vi "Swerve_Wheel.vi"(3 "Kp":dbl, 4 "Offset_Y":dbl, 5 "Offset_X":dbl, 6 "Wheel_Angle":dbl, 7 "Z":dbl, 8 "Y":dbl, 9 "X":dbl) -> (0 "Wheel_Speed":dbl, 1 "Turn_Speed":dbl, 2 "Angle_Goal":dbl)   [LabVIEW 2018]
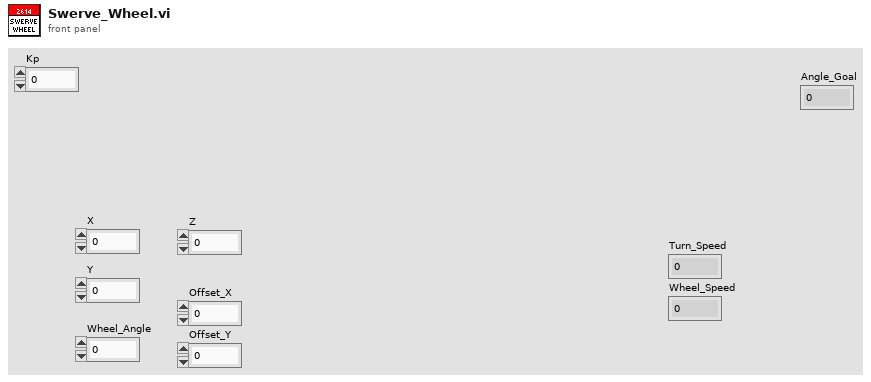
[diagram p1: front panel]
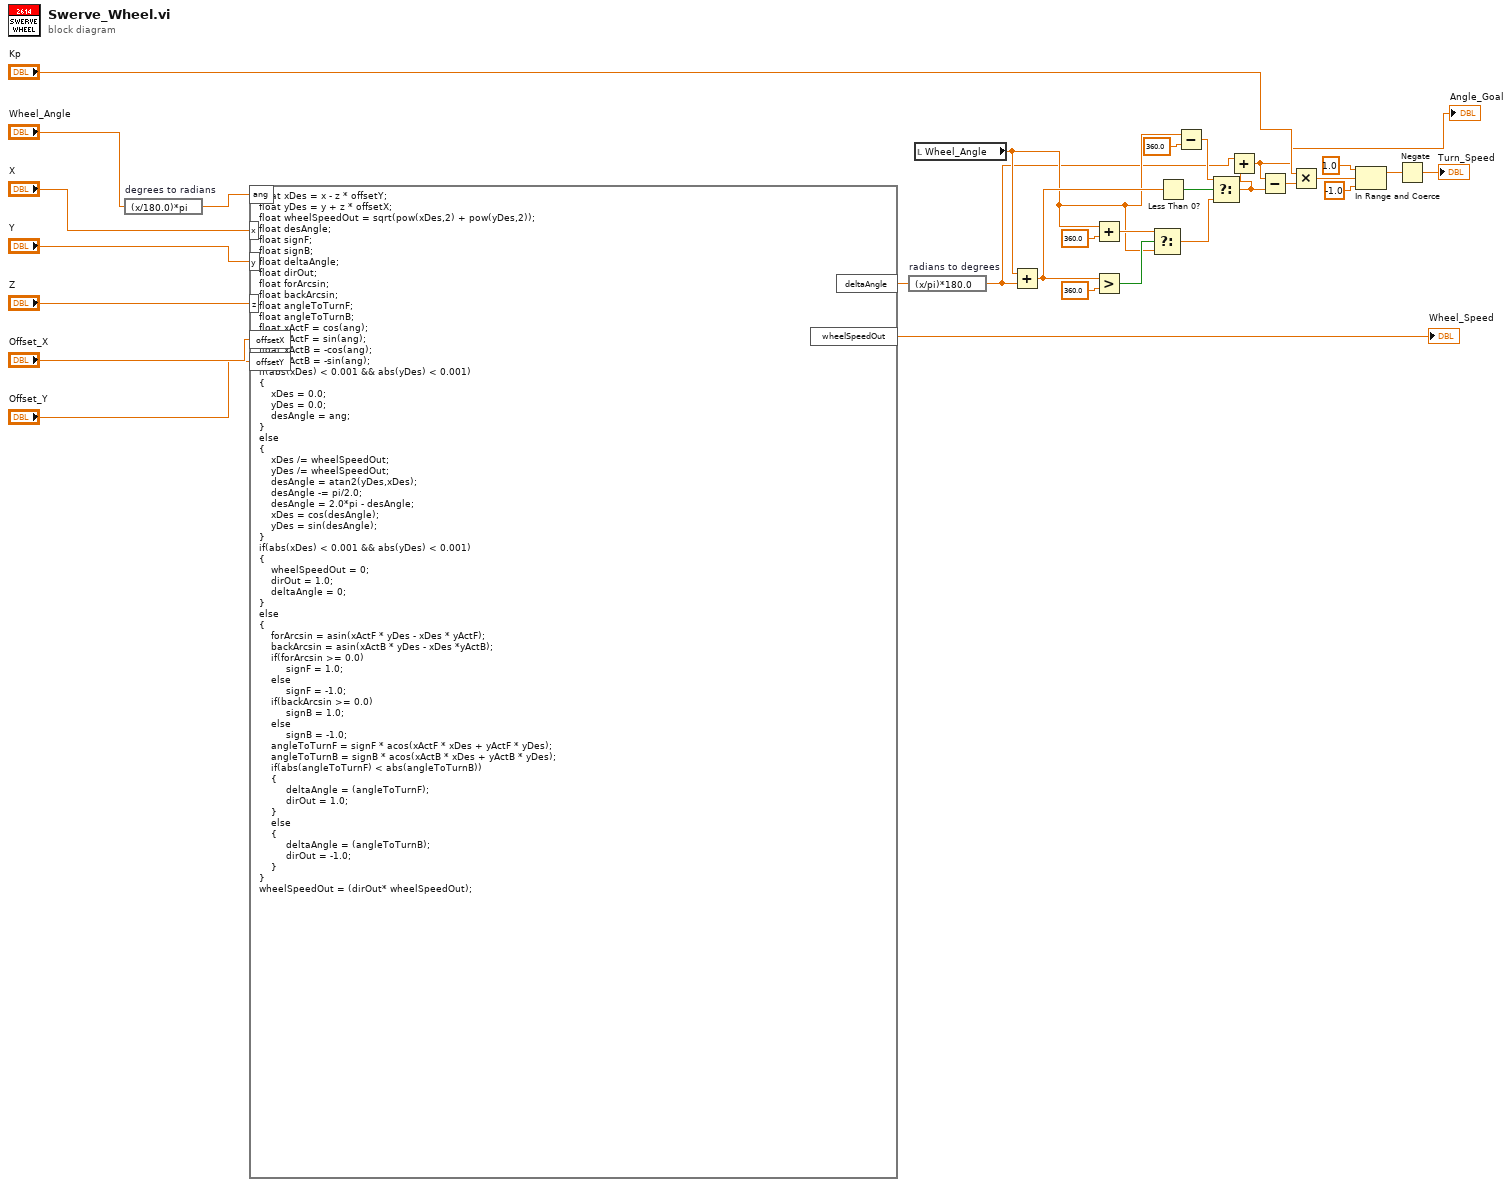
[diagram p0: block diagram]
diagram:
  n1 = expression code="(x/180.0)*pi" "degrees to radians"("Wheel_Angle") -> (w20:dbl)
  n2 = formula code="float xDes = x - z * offsetY;\nfloat yDes = y + z * offsetX;\nfloat wheelSpeedOut = sqrt(pow(xDes,2) + pow(yDes,2));\nfloat desAngle;\nfloat signF;\nfloat signB;\nfloat deltaAngle;\nfloat dirOut;\nfloat forArcsin;\nfloat backArcsin;\nfloat angleToTurnF;\nfloat angleToTurnB;\nfloat xActF = cos(ang);\nfloat yActF = sin(ang);\nfloat xActB = -cos(ang);\nfloat yActB = -sin(ang);\nif(abs(xDes) < 0.001 && abs(yDes) < 0.001)\n{\n    xDes = 0.0;\n    yDes = 0.0;\n    desAngle = ang;\n}\nelse\n{\n    xDes /= wheelSpeedOut;\n    yDes /= wheelSpeedOut;\n    desAngle = atan2(yDes,xDes);\n    desAngle -= pi/2.0;\n    desAngle = 2.0*pi - desAngle;\n    xDes = cos(desAngle);\n    yDes = sin(desAngle);\n}\nif(abs(xDes) < 0.001 && abs(yDes) < 0.001)\n{\n    wheelSpeedOut = 0;\n    dirOut = 1.0;\n    deltaAngle = 0;\n}\nelse\n{\n    forArcsin = asin(xActF * yDes - xDes * yActF);\n    backArcsin = asin(xActB * yDes - xDes *yActB);\n    if(forArcsin >= 0.0)\n         signF = 1.0;\n    else\n         signF = -1.0;\n    if(backArcsin >= 0.0)\n         signB = 1.0;\n    else\n         signB = -1.0;\n    angleToTurnF = signF * acos(xActF * xDes + yActF * yDes);\n    angleToTurnB = signB * acos(xActB * xDes + yActB * yDes);\n    if(abs(angleToTurnF) < abs(angleToTurnB))\n    {\n         deltaAngle = (angleToTurnF);\n         dirOut = 1.0;\n    }\n    else\n    {\n         deltaAngle = (angleToTurnB);\n         dirOut = -1.0;\n    }\n}\nwheelSpeedOut = (dirOut* wheelSpeedOut);"("x"="X", "y"="Y", "ang"=w20, "offsetX"="Offset_X", "z"="Z", "offsetY"="Offset_Y") -> ("wheelSpeedOut"=→"Wheel_Speed":dbl, "deltaAngle"=w9:dbl)
  n3 = expression code="(x/pi)*180.0" "radians to degrees"(w9) -> (w5:dbl)
  n4 = local read "Wheel_Angle"() -> (w8:dbl)
  n5 = Add(x=w8, y=w5) -> (x+y=w16:dbl)
  n6 = Add(x=w8, y=360.0) -> (x+y=w14:dbl)
  n7 = Greater?(x=w16, y=360.0) -> (0:w17:bool)
  n8 = Select(t=w14, s=w17, f=w8) -> (s? t:f=w18:dbl)
  n9 = Less Than 0?(x=w16) -> (x < 0?=w19:bool)
  n10 = Subtract(x=w8, y=360.0) -> (x-y=w11:dbl)
  n11 = Select(t=w11, s=w19, f=w18) -> (s? t:f=w6:dbl)
  n12 = Add(x=w5, y=w6) -> (x+y=w4:dbl)
  "Angle_Goal" <- w4
  n13 = Subtract(x=w4, y=w6) -> (x-y=w12:dbl)
  n14 = Multiply(x="Kp", y=w12) -> (x*y=w25:dbl)
  n15 = In Range and Coerce(upper limit=1.0, x=w25, lower limit=-1.0) -> (coerced(x)=w2:dbl)  [unwired: 1 out]
  n16 = Negate(x=w2) -> (-x=→"Turn_Speed":dbl)
